vi "Initialize.vi"(8 "error in (no error)":errorcluster, 9 "Reset (True)":bool=TRUE, 10 "ID Query (True)":bool=TRUE, 11 "VISA resource name":refnum<visa-resource-name>) -> (0 "error out":errorcluster, 3 "VISA resource name out":refnum<visa-resource-name>)   [LabVIEW 2017, in "Keysight N8900 Series.lvlib"]
doc: "Establishes communication with the instrument and optionally performs an instrument identification query and/or an instrument reset. It also places the instrument in a default state needed for other instrument driver operations. Therefore, call this VI before calling other instrument driver VIs for this instrument. Generally, you need to call the Initialize VI only once at the beginning of an application."
uses:
  Keysight N8900 Series.lvlib
panel:
  # "(c) 2014 National Instruments.  ALL RIGHTS RESERVED."
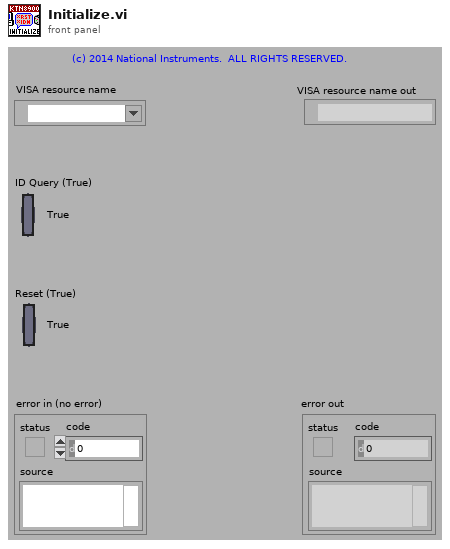
[diagram p1: front panel]
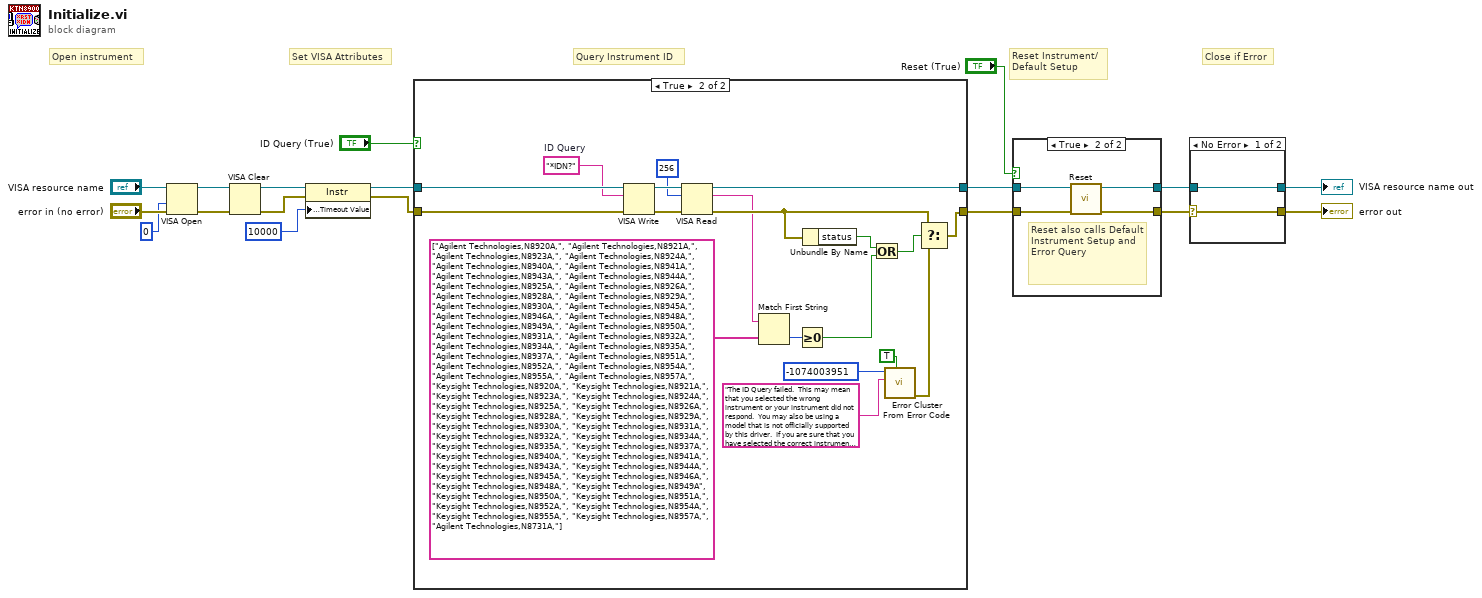
[diagram p0: block diagram]
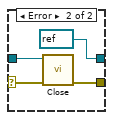
[diagram p2: hidden frame]
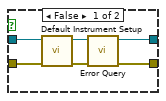
[diagram p3: hidden frame]
diagram:
  # "Set VISA Attributes"
  # "Close if Error"
  # "Query Instrument ID"
  # "Reset Instrument/\nDefault Setup"
  # "Open instrument"
  n1 = VISA Open(access mode=u32 0, error in (no error)="error in (no error)", VISA resource name="VISA resource name") -> (VISA resource name=w10:refnum<visa-resource-name>, error out=w9:errorcluster)  [unwired: 2 in]
  n2 = VISA Clear(VISA resource name=w10, error in (no error)=w9) -> (VISA resource name out=w8:refnum<visa-resource-name>, error out=w7:errorcluster)
  n3 = property class="Instr"(reference=w8, error in=w7, "General Settings:Timeout Value"=u32 10000) -> (reference out=w2:refnum<visa-resource-name>, error out=w1:errorcluster)
  n4 = case shown="True" "ID Query (True)" {
    tunnel: [w19 w39] -> w17
    tunnel: [w20 w36] -> w18
    tunnel: w2 -> [w20 w37]
    tunnel: w1 -> [w19 w38]
    frame False {
    }
    frame True {
      w32 = "*IDN?"  # ID Query
      n5 = VISA Write(VISA resource name=w37, write buffer=w32, error in (no error)=w38) -> (VISA resource name out=w35:refnum<visa-resource-name>, error out=w34:errorcluster)  [unwired: 1 out]
      n6 = VISA Read(VISA resource name=w35, byte count=u32 256, error in (no error)=w34) -> (VISA resource name out=w36:refnum<visa-resource-name>, read buffer=w22:string, error out=w27:errorcluster)  [unwired: 1 out]
      n7 = Match First String(2:string[] ["Agilent Technologies,N8920A,", "Agilent Technologies,N8921A,", "Agilent Technologies,N8923A,", "Agilent Technologies,N8924A,", "Agilent Technologies,N8940A,", "Agilent Technologies,N8941A,", "Agilent Technologies,N8943A,", "Agilent Technologies,N8944A,", "Agilent Technologies,N8925A,", "Agilent Technologies,N8926A,", "Agilent Technologies,N8928A,", "Agilent Technologies,N8929A,", "Agilent Technologies,N8930A,", "Agilent Technologies,N8945A,", "Agilent Technologies,N8946A,", "Agilent Technologies,N8948A,", "Agilent Technologies,N8949A,", "Agilent Technologies,N8950A,", "Agilent Technologies,N8931A,", "Agilent Technologies,N8932A,", "Agilent Technologies,N8934A,", "Agilent Technologies,N8935A,", "Agilent Technologies,N8937A,", "Agilent Technologies,N8951A,", "Agilent Technologies,N8952A,", "Agilent Technologies,N8954A,", "Agilent Technologies,N8955A,", "Agilent Technologies,N8957A,", "Keysight Technologies,N8920A,", "Keysight Technologies,N8921A,", "Keysight Technologies,N8923A,", "Keysight Technologies,N8924A,", "Keysight Technologies,N8925A,", "Keysight Technologies,N8926A,", "Keysight Technologies,N8928A,", "Keysight Technologies,N8929A,", "Keysight Technologies,N8930A,", "Keysight Technologies,N8931A,", "Keysight Technologies,N8932A,", "Keysight Technologies,N8934A,", "Keysight Technologies,N8935A,", "Keysight Technologies,N8937A,", "Keysight Technologies,N8940A,", "Keysight Technologies,N8941A,", "Keysight Technologies,N8943A,", "Keysight Technologies,N8944A,", "Keysight Technologies,N8945A,", "Keysight Technologies,N8946A,", "Keysight Technologies,N8948A,", "Keysight Technologies,N8949A", "Keysight Technologies,N8950A,", "Keysight Technologies,N8951A,", "Keysight Technologies,N8952A,", "Keysight Technologies,N8954A,", "Keysight Technologies,N8955A,", "Keysight Technologies,N8957A,", "Agilent Technologies,N8731A,"] ("string array"), 3:w22) -> (0:w21:i32)  [unwired: 1 out]
      n8 = Greater Or Equal To 0?(x=w21) -> (x >= 0?=w25:bool)
      n9 = Unbundle By Name(w27) -> ("status"=w26:bool)
      n10 = Or(x=w26, y=w25) -> (x .or. y?=w24:bool)
      n11 = call <vilib>:"Error Cluster From Error Code.vi"("show call chain? (False)"=TRUE, "error message (\"\")"="The ID Query failed.  This may mean that you selected the wrong instrument or your instrument did not respond.  You may also be using a model that is not officially supported by this driver.  If you are sure that you have selected the correct instrument and it is responding, try disabling the ID Query." ("Source (VI Name)"), "error code (0)"=-1074003951 ("Code")) -> ("error out"=w31:errorcluster)  [unwired: 6 in]
      n12 = Select(t=w27, s=w24, f=w31) -> (s? t:f=w39:errorcluster)
    }
  }
  n13 = case shown="True" "Reset (True)" {
    tunnel: w17 -> [w44 w46]
    tunnel: [w41 w49] -> w3
    tunnel: w18 -> [w45 w47]
    tunnel: [w42 w48] -> w4
    frame False {
      n14 = call "Default Instrument Setup.vi"("error in (no error)"=w44, "VISA resource name"=w45) -> ("error out"=w40:errorcluster, "VISA resource name out"=w43:refnum<visa-resource-name>)  [unwired: 8 in]
      n15 = call "Error Query.vi"("error in (no error)"=w40, "VISA resource name"=w43) -> ("error out"=w41:errorcluster, "VISA resource name out"=w42:refnum<visa-resource-name>)  [unwired: 6 in, 2 out]
    }
    frame True {
      # "Reset also calls Default Instrument Setup and Error Query"
      n16 = call "Reset.vi"("error in (no error)"=w46, "VISA resource name"=w47) -> ("error out"=w49:errorcluster, "VISA resource name out"=w48:refnum<visa-resource-name>)  [unwired: 8 in]
    }
  }
  n17 = case shown="No Error" w3 {
    selector: w3 -> [w50 w53]
    tunnel: w4 -> [w51 w54]
    tunnel: [w51 refnum<visa-resource-name> refnum ("VISA resource name out")] -> w6
    tunnel: [w50 w55] -> w5
    frame No Error {
    }
    frame Error {
      n18 = call "Close.vi"("error in (no error)"=w53, "VISA resource name"=w54) -> ("error out"=w55:errorcluster)  [unwired: 9 in]
    }
  }
  "VISA resource name out" <- w6
  "error out" <- w5
